vi "validate.vi"(8 "error in":errorcluster, 11 "FPGA Channel configuration in":refnum<class "FPGA Channel configuration.lvclass">) -> (0 "error out":errorcluster, 3 "FPGA Channel configuration out":refnum<class "FPGA Channel configuration.lvclass">)   [LabVIEW 2025, in "FPGA.lvlib" / "FPGA Channel configuration.lvclass"]
doc: "Provides an interface for performing validation on a given configuration. Any children should define the behavior of this function to ensure that the configuration in memory can be used by the runtime class.Copyright 2017 National Instruments Corporation\n\nLicensed under the Apache License, Version 2.0 (the \"License\"); you may not use this file except in compliance with the License. You may obtain a copy of the License at http://www.apache.org/licenses/LICENSE-2.0\nUnless required by applicable law or agreed to in writing, software distributed under the License is distributed on an \"AS IS\" BASIS, WITHOUT WARRANTIES OR CONDITIONS OF ANY KIND, either express or implied. See the License for the specific language governing permissions and limitations under the License."
uses:
  FPGA Channel configuration.lvclass
  FPGA Channel configuration.lvclass/FPGA Channel configuration.ctl
  Users/Public/Documents/Sandia National Labs/TSS Plugin/CEF.lvlibp
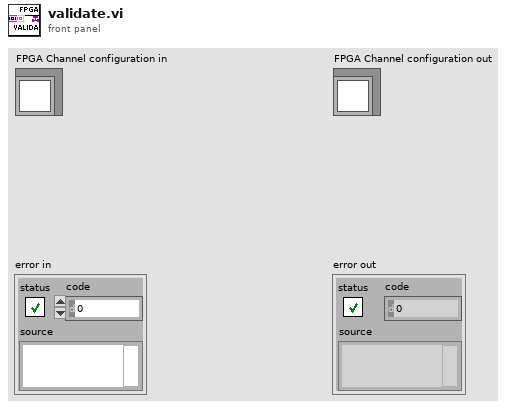
[diagram p1: front panel]
types:
  T1 = cluster{"Address":string, "SW Alias":string, "Enabled":bool, "Type":string, "Description":string}
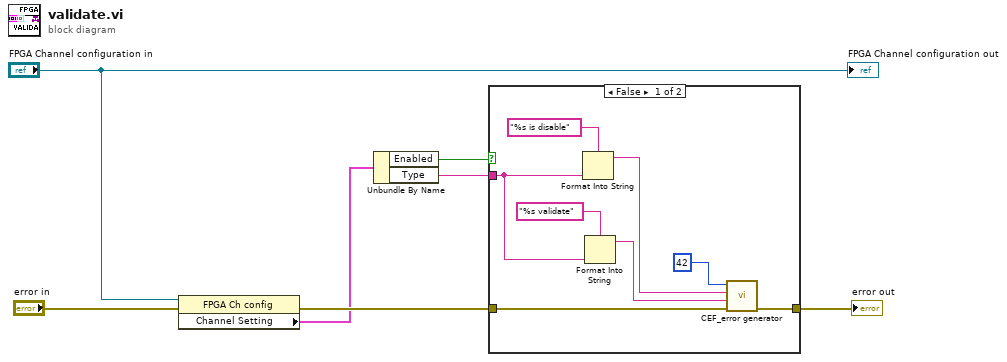
[diagram p0: block diagram]
diagram:
  n1 = property class="FPGA Ch config"(reference="FPGA Channel configuration in", error in="error in") -> (error out=w3:errorcluster, "Channel Setting"=w1:T1)  [unwired: 1 out]
  n2 = Unbundle By Name(w1) -> ("Enabled"=w7:bool, "Type"=w4:string)
  n3 = case shown="False" w7 {
    tunnel: w3 -> [w15 w16]
    tunnel: [w14 w16] -> w5
    tunnel: w4 -> [w9 _]
    frame False {
      n4 = Format Into String(format string="%s is disable" ("append error message"), w9) -> (resulting string=w11:string)  [unwired: 2 in, 1 out]
      n5 = Format Into String(format string="%s validate" ("append error message"), w9) -> (resulting string=w8:string)  [unwired: 2 in, 1 out]
      n6 = call "CEF_error generator.vi"("error in"=w15, "source"=w8, "append error message"=w11, "error code (0)"=42) -> ("error out"=w14:errorcluster)  [unwired: 5 in]
    }
    frame True {
    }
  }
  "error out" <- w5
  "FPGA Channel configuration out" <- "FPGA Channel configuration in"
